vi "修改游标线宽.vi"(10 "活动游标":u32, 11 "XYGraph输入":refnum<vi>) -> ()   [LabVIEW 2015]
uses:
  GlobalVariables.vi
panel:
  out "游标.线条宽度old":u8
  in  "取消":bool caption="查看所有值表"
  in  "确定":bool caption="查看所有值表"
  in  "线宽选项":u8(ring) items=["特细", "细", "中", "粗", "特粗"]
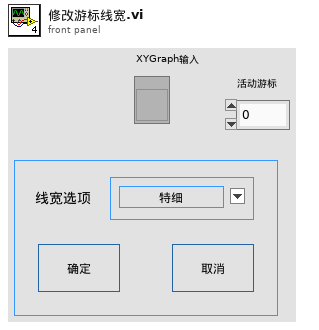
[diagram p1: front panel]
types:
  T1 = cluster{"Visible":bool, "Color":u32, "LineWidth":u8}
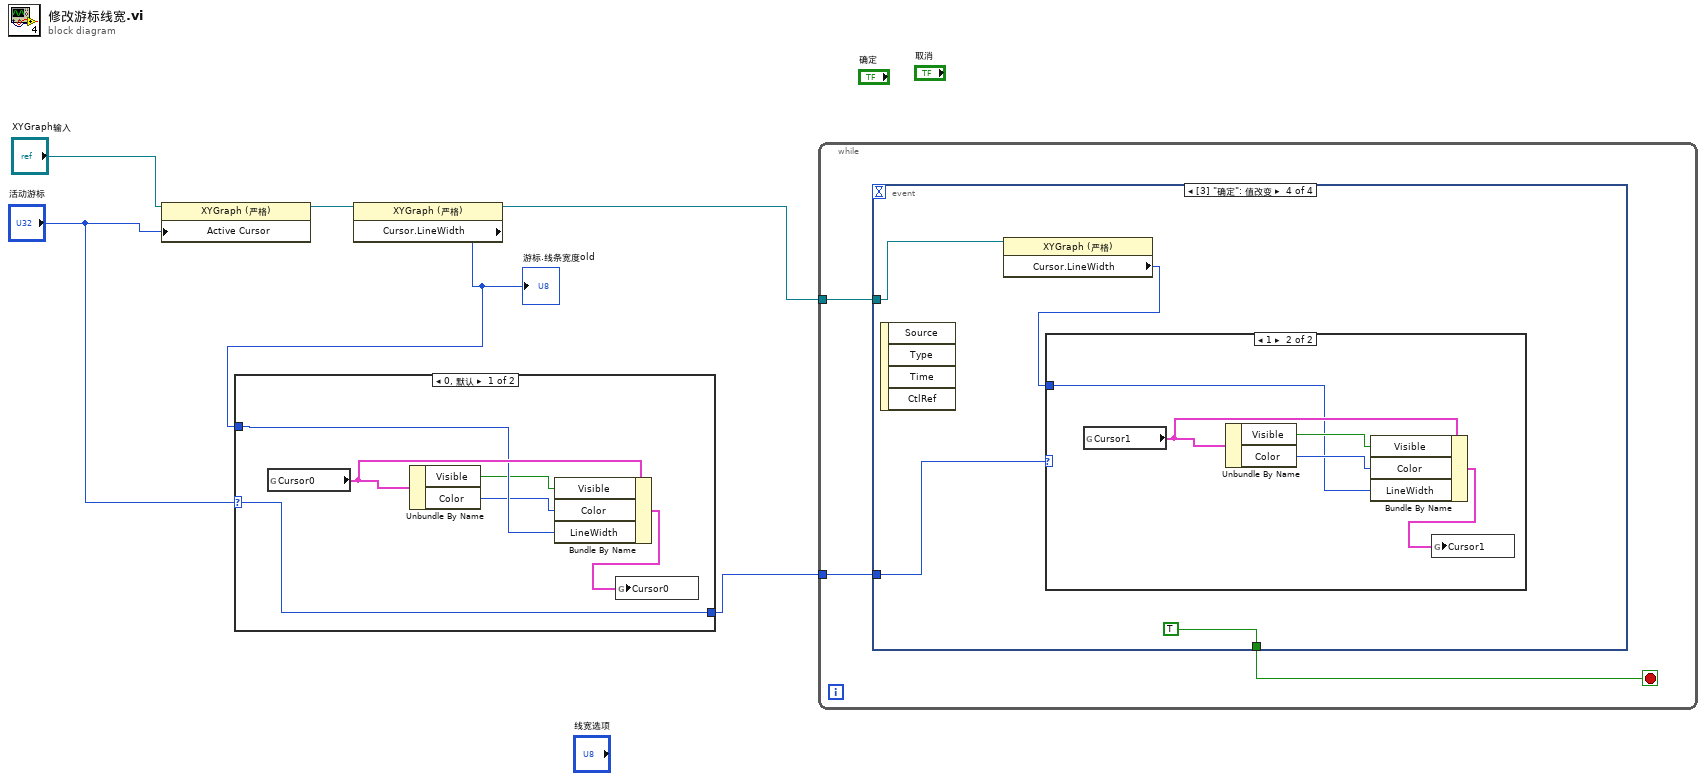
[diagram p0: block diagram]
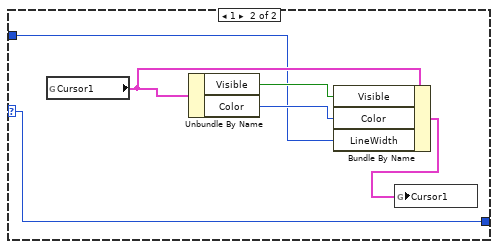
[diagram p2: hidden frame]
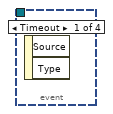
[diagram p3: hidden frame]
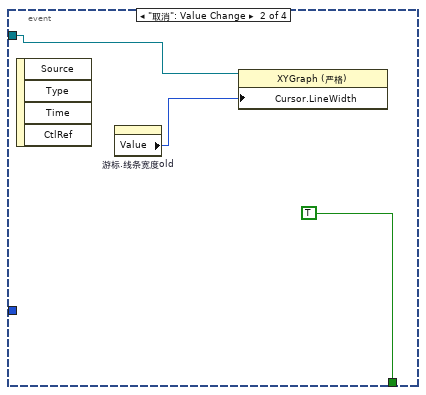
[diagram p4: hidden frame]
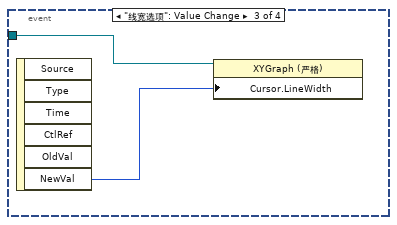
[diagram p5: hidden frame]
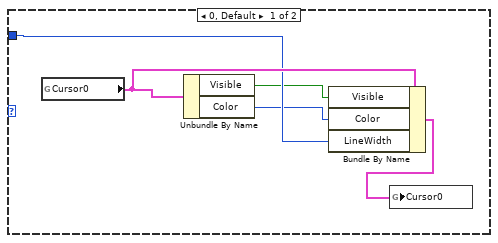
[diagram p6: hidden frame]
diagram:
  n1 = property class="XYGraph (严格)"(reference="XYGraph输入", "Active Cursor"="活动游标") -> (reference out=w5:refnum<vi>)  [unwired: 1 in, 1 out]
  n2 = property class="XYGraph (严格)"(reference=w5) -> (reference out=w4:refnum<vi>, "Cursor.LineWidth"=w2:u8)  [unwired: 1 in, 1 out]
  "游标.线条宽度old" <- w2
  n3 = case shown="0, 默认" "活动游标" {
    selector: "活动游标" -> [w7 w13]
    tunnel: w2 -> [w11 w14]
    tunnel: [w7 w13] -> w1
    frame 0, Default {
      n4 = global read "GlobalVariables.vi" "Cursor0"() -> (w12:T1)
      n5 = Unbundle By Name(w12) -> ("Visible"=w10:bool, "Color"=w9:u32)
      n6 = Bundle By Name(cluster=w12, "Visible"=w10, "Color"=w9, "LineWidth"=w11) -> (w8:T1)
      n7 = global write "GlobalVariables.vi" "Cursor0"(w8) -> ()
    }
    frame 1 {
      n8 = global read "GlobalVariables.vi" "Cursor1"() -> (w18:T1)
      n9 = Unbundle By Name(w18) -> ("Visible"=w17:bool, "Color"=w16:u32)
      n10 = Bundle By Name(cluster=w18, "Visible"=w17, "Color"=w16, "LineWidth"=w14) -> (w15:T1)
      n11 = global write "GlobalVariables.vi" "Cursor1"(w15) -> ()
    }
  }
  n12 = while {
    tunnel: w4 -> [w20]
    tunnel: w1 -> [w19]
    stop <- w21 stop-if-true
    n13 = event shown="[3] \"确定\": 值改变" {
      selector: _ -> [_ _ _ _]
      dyn-events: _ -> [_ _ _ _]
      timeout: _ -> [_ _ _ _]
      tunnel: [_ TRUE _ TRUE] -> w21
      tunnel: w20 -> [_ w24 w26 w29]
      tunnel: w19 -> [_ _ _ w27]
      event Timeout {
        n14 = event-data() -> ()  [unwired: 1 in, 2 out]
      }
      event "取消": Value Change {
        n15 = event-data() -> ()  [unwired: 1 in, 4 out]
        n16 = property on="游标.线条宽度old" class="DigNum (严格)"() -> ("Value"=w23:u8)  [unwired: 2 in, 2 out]
        n17 = property class="XYGraph (严格)"(reference=w24, "Cursor.LineWidth"=w23) -> ()  [unwired: 1 in, 2 out]
      }
      event "线宽选项": Value Change {
        n18 = event-data() -> ("NewVal"=w25:u8)  [unwired: 1 in, 5 out]
        n19 = property class="XYGraph (严格)"(reference=w26, "Cursor.LineWidth"=w25) -> ()  [unwired: 1 in, 2 out]
      }
      event "确定": Value Change {
        n20 = event-data() -> ()  [unwired: 1 in, 4 out]
        n21 = property class="XYGraph (严格)"(reference=w29) -> ("Cursor.LineWidth"=w28:u8)  [unwired: 1 in, 2 out]
        n22 = case shown="1" w27 {
          tunnel: w28 -> [w34 w36]
          frame 0, Default {
            n23 = global read "GlobalVariables.vi" "Cursor0"() -> (w35:T1)
            n24 = Unbundle By Name(w35) -> ("Visible"=w33:bool, "Color"=w32:u32)
            n25 = Bundle By Name(cluster=w35, "Visible"=w33, "Color"=w32, "LineWidth"=w34) -> (w31:T1)
            n26 = global write "GlobalVariables.vi" "Cursor0"(w31) -> ()
          }
          frame 1 {
            n27 = global read "GlobalVariables.vi" "Cursor1"() -> (w40:T1)
            n28 = Unbundle By Name(w40) -> ("Visible"=w39:bool, "Color"=w38:u32)
            n29 = Bundle By Name(cluster=w40, "Visible"=w39, "Color"=w38, "LineWidth"=w36) -> (w37:T1)
            n30 = global write "GlobalVariables.vi" "Cursor1"(w37) -> ()
          }
        }
      }
    }
  }
